vi "GoToWavelength.vi"(8 "error in (no error)":errorcluster, 10 "Wavelength":dbl, 11 "HRS_Spectrometer in":refnum<class "HRS_Spectrometer.lvclass">) -> (0 "error out":errorcluster, 3 "HRS_Spectrometer out":refnum<class "HRS_Spectrometer.lvclass">)   [LabVIEW 2023, in "Spectrometer Library.lvlib" / "HRS_Spectrometer.lvlib" / "HRS_Spectrometer.lvclass"]
uses:
  HRS_Spectrometer.lvclass
  HRS_Spectrometer.lvclass/HRS_Spectrometer.ctl
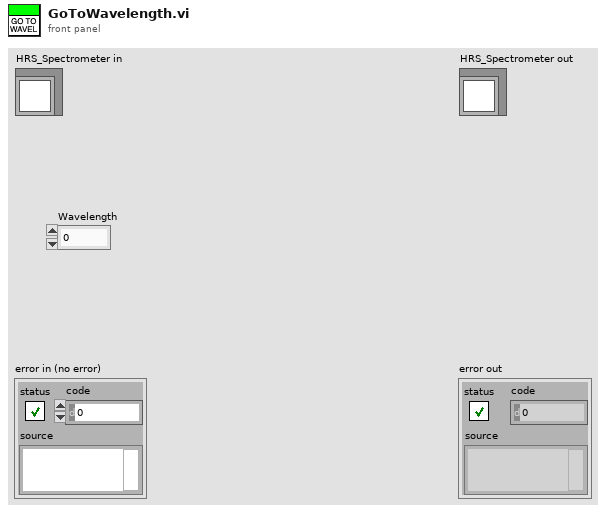
[diagram p1: front panel]
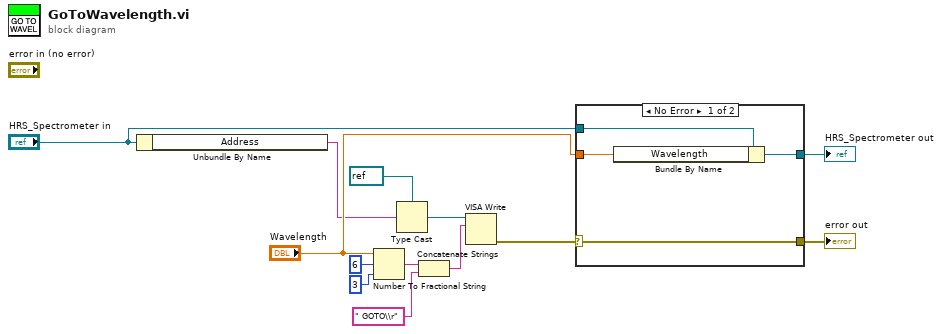
[diagram p0: block diagram]
diagram:
  n1 = Unbundle By Name("HRS_Spectrometer in") -> ("Address"=w3:string)
  n2 = Number To Fractional String(number="Wavelength", width (-)=i16 6, precision (6)=i16 3) -> (F-format string=w7:string)  [unwired: 1 in]
  n3 = Type Cast(type=refnum<visa-resource-name> refnum ("VISA resource name"), x=w3) -> (*(type *) &x=w2:refnum<visa-resource-name>)
  n4 = Concatenate Strings(w7, " GOTO\\r") -> (w6:string)
  n5 = VISA Write(VISA resource name=w2, write buffer=w6) -> (error out=w1:errorcluster)  [unwired: 1 in, 2 out]
  n6 = case shown="No Error" w1 {
    selector: w1 -> [w14 w18]
    tunnel: "HRS_Spectrometer in" -> [w17 w19]
    tunnel: "Wavelength" -> [w16 _]
    tunnel: [w15 w19] -> w10
    tunnel: [w14 w18] -> w5
    frame No Error {
      n7 = Bundle By Name(cluster=w17, "Wavelength"=w16) -> (w15:refnum<class "HRS_Spectrometer.lvclass">)
    }
    frame Error {
    }
  }
  "error out" <- w5
  "HRS_Spectrometer out" <- w10
